vi "FileAppenderConfigDTOFromNative.vi"(8 "error in (no error)":errorcluster, 11 "FileAppenderConfig":T1={"common"={"id"="", "threshold"=enum."INFO", "filter"={"mode"=enum."Mirror", "levelMin"=enum."INFO", "levelMax"=enum."INFO", "tagPrefix"=""}, "queueBound"=0, "dropPolicy"=enum."DropOldest"}, "rootFolder"=path "", "maxFileSize"=0, "maxFileCount"=0, "baseName"="", "extension"="", "delimiter"="", "calendarFolderTree"=FALSE, "useUTC"=FALSE}) -> (0 "error out":errorcluster, 3 "FileAppenderConfigDTO":T7={"common"={"id"="", "threshold"="INFO", "filter"={"mode"="Mirror", "levelMin"="INFO", "levelMax"="INFO", "tagPrefix"=""}, "queueBound"=0, "dropPolicy"="DropOldest"}, "rootFolder"="", "maxFileSize"=0, "maxFileCount"=0, "baseName"="", "extension"="", "delimiter"="", "calendarFolderTree"=FALSE, "useUTC"=FALSE})   [LabVIEW 2026, in "Lumberjack.lvlib"]
uses:
  Lumberjack.lvlib
  TypeDefs/ConfigDTO/FilterDTO.ctl
  TypeDefs/ConfigDTO/AppenderConfigDTO.ctl
  TypeDefs/ConfigDTO/FileAppenderConfigDTO.ctl
  TypeDefs/Severity.ctl
  TypeDefs/FilterMode.ctl
  TypeDefs/Filter.ctl
  TypeDefs/DropPolicy.ctl
  TypeDefs/AppenderConfig.ctl
  TypeDefs/FileAppenderConfig.ctl
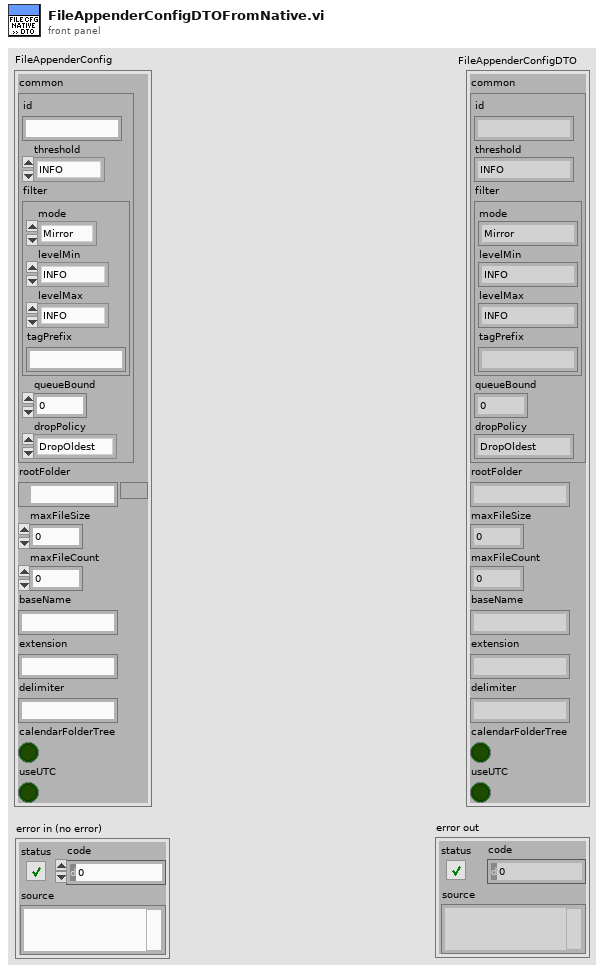
[diagram p1: front panel]
types:
  T1 = typedef "Lumberjack.lvlib/FileAppenderConfig.ctl" = cluster{"common":T2, "rootFolder":path, "maxFileSize":i64, "maxFileCount":i32, "baseName":string, "extension":string, "delimiter":string, "calendarFolderTree":bool, "useUTC":bool}
  T2 = typedef "Lumberjack.lvlib/AppenderConfig.ctl" = cluster{"id":string, "threshold":T3, "filter":T4, "queueBound":i32, "dropPolicy":T6}
  T3 = typedef "Lumberjack.lvlib/Severity.ctl" = enum16{"OFF", "FATAL", "ERROR", "WARN", "INFO", "DEBUG", "TRACE", "ALL"}
  T4 = typedef "Lumberjack.lvlib/Filter.ctl" = cluster{"mode":T5, "levelMin":T3, "levelMax":T3, "tagPrefix":string}
  T5 = typedef "Lumberjack.lvlib/FilterMode.ctl" = enum16{"Mirror", "Routed"}
  T6 = typedef "Lumberjack.lvlib/DropPolicy.ctl" = enum16{"DropOldest", "DropNewest", "LevelAware"}
  T7 = typedef "Lumberjack.lvlib/FileAppenderConfigDTO.ctl" = cluster{"common":T8, "rootFolder":string, "maxFileSize":i64, "maxFileCount":i32, "baseName":string, "extension":string, "delimiter":string, "calendarFolderTree":bool, "useUTC":bool}
  T8 = typedef "Lumberjack.lvlib/AppenderConfigDTO.ctl" = cluster{"id":string, "threshold":string, "filter":T9, "queueBound":i32, "dropPolicy":string}
  T9 = typedef "Lumberjack.lvlib/FilterDTO.ctl" = cluster{"mode":string, "levelMin":string, "levelMax":string, "tagPrefix":string}
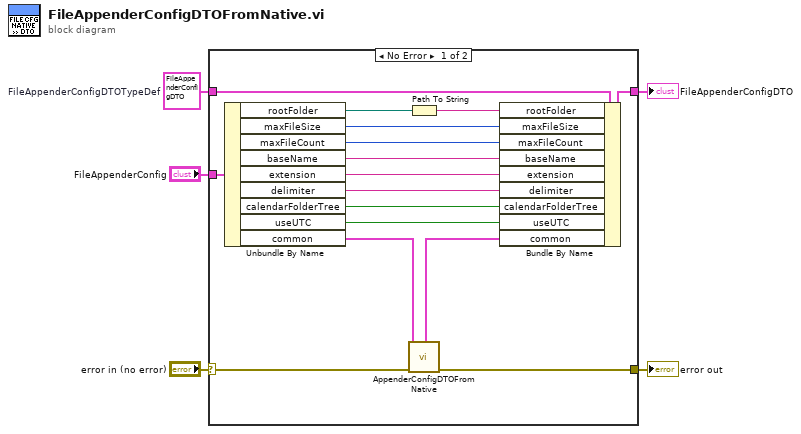
[diagram p0: block diagram]
diagram:
  w3 = T7 {"common"={"id"="", "threshold"="INFO", "filter"={"mode"="Mirror", "levelMin"="INFO", "levelMax"="INFO", "tagPrefix"=""}, "queueBound"=0, "dropPolicy"="DropOldest"}, "rootFolder"="", "maxFileSize"=0, "maxFileCount"=0, "baseName"="", "extension"="", "delimiter"="", "calendarFolderTree"=FALSE, "useUTC"=FALSE}  # FileAppenderConfigDTOTypeDef
  n1 = case shown="No Error" "error in (no error)" {
    selector: "error in (no error)" -> [w21 w23]
    tunnel: [w18 w23] -> w1
    tunnel: "FileAppenderConfig" -> [w19 _]
    tunnel: [w20 w22] -> w2
    tunnel: w3 -> [w17 w22]
    frame No Error {
      n2 = Unbundle By Name(w19) -> ("rootFolder"=w16:path, "maxFileSize"=w14:i64, "maxFileCount"=w13:i32, "baseName"=w12:string, "extension"=w11:string, "delimiter"=w10:string, "calendarFolderTree"=w9:bool, "useUTC"=w8:bool, "common"=w7:T2)
      n3 = Path To String(path=w16) -> (string=w15:string)
      n4 = call "AppenderConfigDTOFromNative.vi"("error in (no error)"=w21, "AppenderConfig"=w7) -> ("error out"=w18:errorcluster, "AppenderConfigDTO"=w6:T8)  [unwired: 8 in]
      n5 = Bundle By Name(cluster=w17, "rootFolder"=w15, "maxFileSize"=w14, "maxFileCount"=w13, "baseName"=w12, "extension"=w11, "delimiter"=w10, "calendarFolderTree"=w9, "useUTC"=w8, "common"=w6) -> (w20:T7)
    }
    frame Error {
    }
  }
  "error out" <- w1
  "FileAppenderConfigDTO" <- w2
